vi "Flatten Pixmap.vi"(4 "mask":u8[](array[numeric]), 6 "colors":u32[](array[numeric]), 7 "top left":cluster{"x":i16, "y":i16}, 8 "1-bit pixmap":bool[][](array[boolean]), 9 "4-bit pixmap":u8[][](array[numeric]), 10 "8-bit pixmap":u8[][](array[numeric]), 11 "24-bit pixmap":u32[][](array[numeric])) -> (2 "image data":T1)   [LabVIEW 2011]
doc: "Converts pixmap data from a 2D array to a 1D array."
uses:
  imagedata.ctl
panel:
  in  "image data":T1
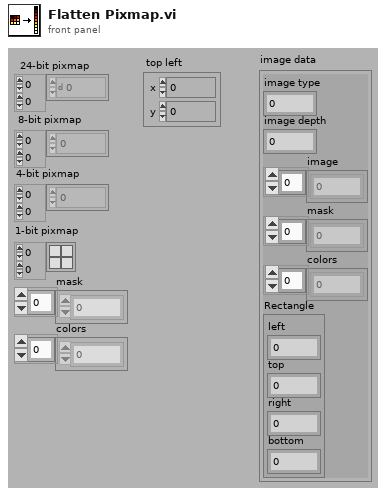
[diagram p1: front panel]
types:
  T1 = typedef "imagedata.ctl" = cluster{"image type":i32, "image depth":i32, "image":u8[], "mask":u8[], "colors":u32[], "Rectangle":cluster{"left":i16, "top":i16, "right":i16, "bottom":i16}}
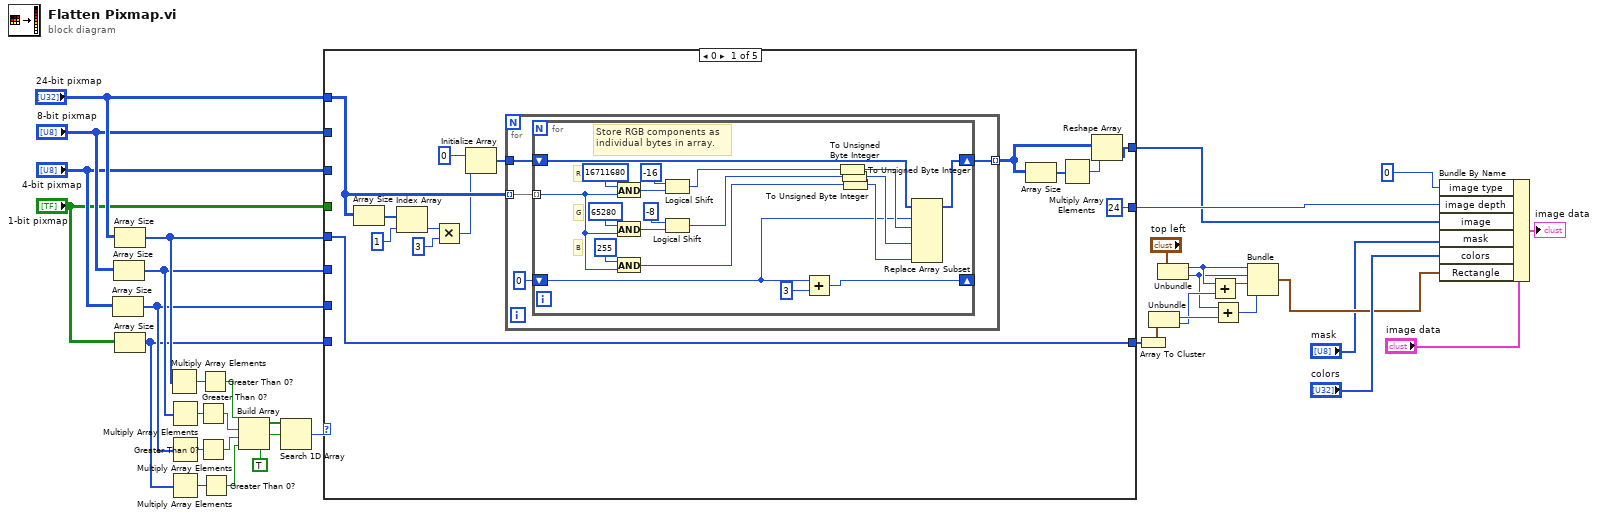
[diagram p0: block diagram]
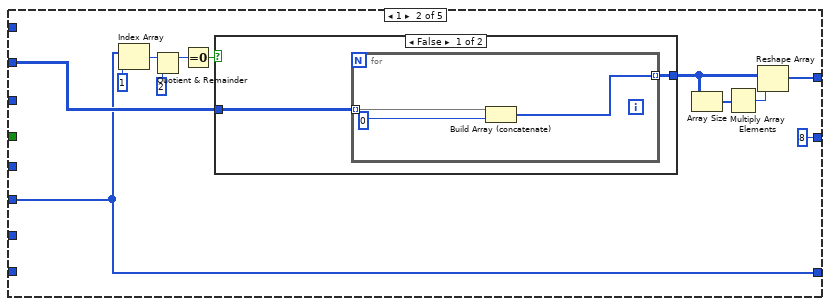
[diagram p2: hidden frame]
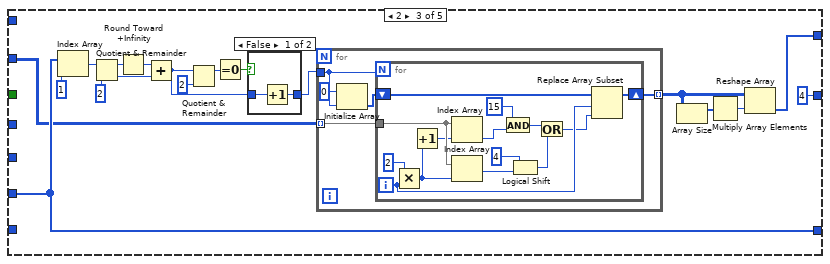
[diagram p4: hidden frame]
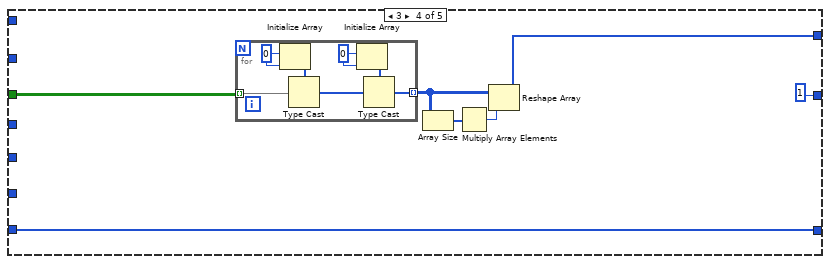
[diagram p6: hidden frame]
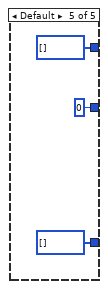
[diagram p7: hidden frame]
diagram:
  n1 = Array Size(array="4-bit pixmap") -> (size(s)=w19:i32[])
  n2 = Array Size(array="8-bit pixmap") -> (size(s)=w20:i32[])
  n3 = Array Size(array="24-bit pixmap") -> (size(s)=w21:i32[])
  n4 = Array Size(array="1-bit pixmap") -> (size(s)=w18:i32[])
  n5 = Multiply Array Elements(1:w21) -> (0:w36:i32)
  n6 = Multiply Array Elements(1:w20) -> (0:w35:i32)
  n7 = Multiply Array Elements(1:w19) -> (0:w34:i32)
  n8 = Multiply Array Elements(1:w18) -> (0:w33:i32)
  n9 = Greater Than 0?(x=w35) -> (x > 0?=w30:bool)
  n10 = Greater Than 0?(x=w34) -> (x > 0?=w29:bool)
  n11 = Greater Than 0?(x=w36) -> (x > 0?=w31:bool)
  n12 = Greater Than 0?(x=w33) -> (x > 0?=w28:bool)
  n13 = Build Array(w31, w30, w29, w28) -> (w32:bool[])
  n14 = Search 1D Array(1D array=w32, element=TRUE) -> (index of element=w26:i32)  [unwired: 1 out]
  n15 = case shown="0" w26 {
    tunnel: [w47 w80 w96 w134 u8[] [] ("8-bit pixmap")] -> w2
    tunnel: "24-bit pixmap" -> [w44 _ _ _ _]
    tunnel: "8-bit pixmap" -> [_ w79 _ _ _]
    tunnel: "4-bit pixmap" -> [_ _ w92 _ _]
    tunnel: "1-bit pixmap" -> [_ _ _ w135 _]
    tunnel: [24 8 4 1 0] -> w6
    tunnel: w21 -> [w45 _ _ _ _]
    tunnel: w20 -> [_ w76 _ _ _]
    tunnel: w19 -> [_ _ w94 _ _]
    tunnel: w18 -> [_ _ _ w132 _]
    tunnel: [w45 w76 w94 w132 i32[] []] -> w17
    frame 0 {
      n16 = Array Size(array=w44) -> (size(s)=w43:i32[])
      n17 = Index Array(array=w43, index=1) -> (element=w41:i32)
      n18 = Multiply(x=w41, y=3) -> (x*y=w39:i32)
      n19 = Initialize Array(u8 0, w39) -> (w37:u8[])
      n20 = for {
        tunnel: w44 -> [w52] mode=indexing
        tunnel: [w54] -> w48 mode=indexing
        tunnel: w37 -> [w51]
        n21 = for {
          tunnel: w52 -> [w63] mode=indexing
          shift-right: [w57] -> w54
          shift-left: w51 -> [w58]
          shift-right: [w56] -> _
          shift-left: 0 -> [w55]
          # "B"
          # "G"
          # "R"
          # "Store RGB components as\nindividual bytes in array."
          n22 = And(x=16711680, y=w63) -> (x .and. y?=w68:u32)
          n23 = And(x=65280, y=w63) -> (x .and. y?=w67:u32)
          n24 = And(x=255, y=w63) -> (x .and. y?=w64:u32)
          n25 = Logical Shift(y=i8 -16, x=w68) -> (x << y=w66:u32)
          n26 = Logical Shift(y=i8 -8, x=w67) -> (x << y=w65:u32)
          n27 = Add(x=w55, y=3) -> (x+y=w56:i32)
          n28 = To Unsigned Byte Integer(number=w66) -> (unsigned 8bit integer=w61:u8)
          n29 = To Unsigned Byte Integer(number=w65) -> (unsigned 8bit integer=w60:u8)
          n30 = To Unsigned Byte Integer(number=w64) -> (unsigned 8bit integer=w59:u8)
          n31 = Replace Array Subset(array=w58, new element #1=w61, index #1=w55, new element #2=w60, new element #3=w59) -> (w57:u8[])  [unwired: 2 in]
        }
      }
      n32 = Array Size(array=w48) -> (size(s)=w49:i32[])
      n33 = Multiply Array Elements(1:w49) -> (0:w50:i32)
      n34 = Reshape Array(w48, w50) -> (w47:u8[])
    }
    frame 1 {
      n35 = Index Array(array=w76, index=1) -> (element=w75:i32)
      n36 = Quotient & Remainder(x=w75, y=2) -> (x-y*floor(x/y)=w81:i32)  [unwired: 1 out]
      n37 = Equal To 0?(x=w81) -> (x = 0?=w78:bool)
      n38 = case shown="False" w78 {
        tunnel: [w86 w91] -> w83
        tunnel: w79 -> [w87 w91]
        frame False {
          n39 = for {
            tunnel: w87 -> [w90] mode=indexing
            tunnel: [w88] -> w86 mode=indexing
            n40 = Build Array (concatenate)(w90, u8 0) -> (w88:u8[])
          }
        }
        frame True {
        }
      }
      n41 = Array Size(array=w83) -> (size(s)=w84:i32[])
      n42 = Multiply Array Elements(1:w84) -> (0:w85:i32)
      n43 = Reshape Array(w83, w85) -> (w80:u8[])
    }
    frame 2 {
      n44 = Index Array(array=w94, index=1) -> (element=w108:i32)
      n45 = Quotient & Remainder(x=w108, y=2) -> (x-y*floor(x/y)=w102:i32, floor(x/y)=w100:i32)
      n46 = Round Toward +Infinity(x=w102) -> (ceil(x): smallest int >= x=w101:i32)
      n47 = Add(x=w101, y=w100) -> (x+y=w99:i32)
      n48 = Quotient & Remainder(x=w99, y=2) -> (x-y*floor(x/y)=w105:i32)  [unwired: 1 out]
      n49 = Equal To 0?(x=w105) -> (x = 0?=w104:bool)
      n50 = case shown="False" w104 {
        tunnel: w99 -> [w111 w112]
        tunnel: [w110 w112] -> w93
        frame False {
          n51 = Increment(x=w111) -> (x+1=w110:i32)
        }
        frame True {
        }
      }
      n52 = for {
        tunnel: w92 -> [w117] mode=indexing
        tunnel: [w116] -> w98 mode=indexing
        tunnel: w93 -> [w114]
        n53 = Initialize Array(u8 0, w114) -> (w113:u8[])
        n54 = for {
          N: w114 -> [_]
          tunnel: w117 -> [w131]
          shift-right: [w121] -> w116
          shift-left: w113 -> [w118]
          i -> [w120]
          n55 = Multiply(x=2, y=w120) -> (x*y=w129:i32)
          n56 = Increment(x=w129) -> (x+1=w128:i32)
          n57 = Index Array(array=w131, index=w128) -> (element=w127:u8)
          n58 = Index Array(array=w131, index=w129) -> (element=w125:u8)
          n59 = And(x=u8 15, y=w127) -> (x .and. y?=w124:u8)
          n60 = Logical Shift(y=u8 4, x=w125) -> (x << y=w123:u8)
          n61 = Or(x=w124, y=w123) -> (x .or. y?=w119:u8)
          n62 = Replace Array Subset(array=w118, new element=w119, index=w120) -> (w121:u8[])
        }
      }
      n63 = Array Size(array=w98) -> (size(s)=w97:i32[])
      n64 = Multiply Array Elements(1:w97) -> (0:w106:i32)
      n65 = Reshape Array(w98, w106) -> (w96:u8[])
    }
    frame 3 {
      n66 = for {
        tunnel: [w142] -> w138 mode=indexing
        tunnel: w135 -> [w139] mode=indexing
        w141 = u8 0
        w144 = i16 0
        n67 = Initialize Array(w144, w144) -> (w145:i16[])
        n68 = Type Cast(type=w145, x=w139) -> (*(type *) &x=w143:i16[])
        n69 = Initialize Array(w141, w141) -> (w140:u8[])
        n70 = Type Cast(type=w140, x=w143) -> (*(type *) &x=w142:u8[])
      }
      n71 = Array Size(array=w138) -> (size(s)=w136:i32[])
      n72 = Multiply Array Elements(1:w136) -> (0:w137:i32)
      n73 = Reshape Array(w138, w137) -> (w134:u8[])
    }
    frame Default {
    }
  }
  n74 = Array To Cluster(array=w17) -> (cluster=w16:cluster{"[0]":i32, "[1]":i32})
  n75 = Unbundle(w16) -> ("[0]"=w15:i32, "[1]"=w12:i32)
  n76 = Unbundle("top left") -> ("x"=w13:i16, "y"=w11:i16)
  n77 = Add(x=w13, y=w12) -> (x+y=w9:i32)
  n78 = Add(x=w11, y=w15) -> (x+y=w10:i32)
  n79 = Bundle("x"=w13, "y"=w11, w9, w10) -> (w4:cluster{"x":i16, "y":i16, i32, i32})  [unwired: 1 out]
  n80 = Bundle By Name(cluster="image data", "image type"=u16 0, "image depth"=w6, "image"=w2, "mask"="mask", "colors"="colors", "Rectangle"=w4) -> (→"image data":T1)
